vi "Lab14.vi"() -> ()   [LabVIEW 2022 SP3]
uses:
  <vilib>/DAQmx/create/channels.llb/DAQmx Create Channel (CO-Pulse Generation-Frequency).vi
  <vilib>/DAQmx/configure/timing.llb/DAQmx Timing (Implicit).vi
  <resource>/objmgr/daqmx.rc
panel:
  in  "Duty Cycle":dbl(slide)=0.01 min=0.01 max=0.99 step=0.01 scale=0.0..1.0
  out "Iteration Number":i32
  in  "CO.Pulse.Term":tag="/Dev1/PFI1"
  in  "stop":bool
  in  "Counter":tag="Dev1/ctr0"
  in  "Frequency":dbl(slide)=5000.0 min=1.0 max=25000000.0 step=1.0 scale=1.0..25000000.0 scale format="%#_6p"
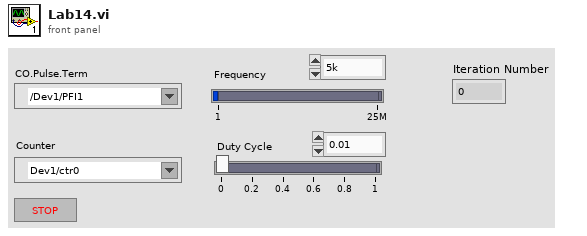
[diagram p1: front panel]
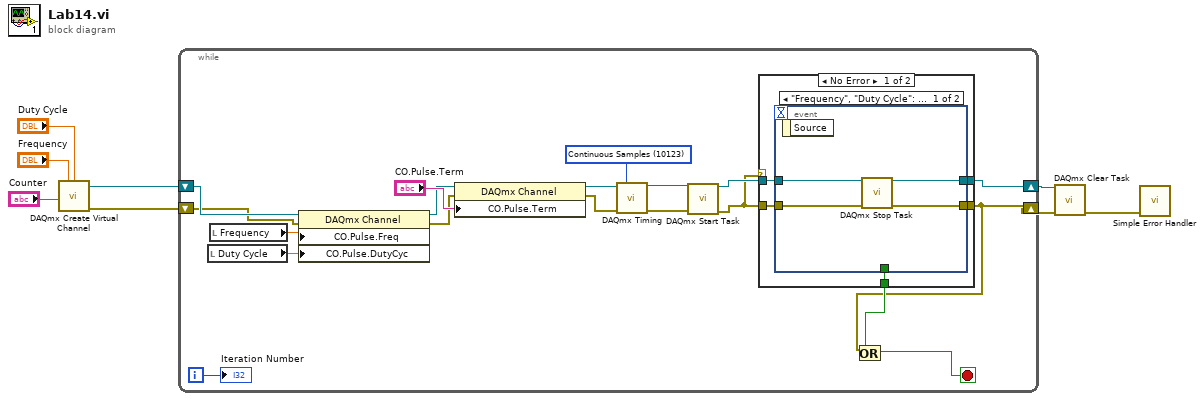
[diagram p0: block diagram]
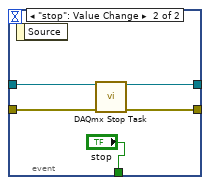
[diagram p2: hidden frame]
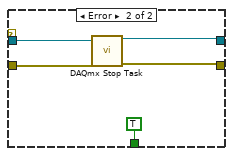
[diagram p3: hidden frame]
diagram:
  n1 = call-poly <vilib>:"DAQmx Create Virtual Channel.vi"("frequency"="Frequency", "duty cycle"="Duty Cycle", "counter"="Counter") -> ("task out"=w5:refnum<k21>, "error out"=w4:errorcluster)  [unwired: 11 in]
  n2 = while {
    shift-right: [w9] -> w2
    shift-left: w4 -> [w17]
    shift-right: [w20] -> w3
    shift-left: w5 -> [w18]
    i -> [w14]
    stop <- w11 stop-if-true
    w21 = 10123 items=["Finite Samples"=10178, "Continuous Samples"=10123, "Hardware Timed Single Point"=12522] ("sample mode")
    n3 = local read "Duty Cycle"() -> (w13:dbl)
    n4 = local read "Frequency"() -> (w19:dbl)
    n5 = property class="DAQmx Channel"(reference=w18, error in=w17, "CO.Pulse.Freq"=w19, "CO.Pulse.DutyCyc"=w13) -> (reference out=w16:refnum<k21>, error out=w15:errorcluster)
    n6 = property class="DAQmx Channel"(reference=w16, error in=w15, "CO.Pulse.Term"="CO.Pulse.Term") -> (reference out=w25:refnum<k21>, error out=w24:errorcluster)
    n7 = call-poly <vilib>:"DAQmx Timing.vi"("task/channels in"=w25, "sample mode"=w21, "error in"=w24) -> ("task out"=w23:refnum<k21>, "error out"=w22:errorcluster)  [unwired: 11 in]
    n8 = call <vilib>:"DAQmx Start Task.vi"("task/channels in"=w23, "error in"=w22) -> ("task out"=w27:refnum<k21>, "error out"=w10:errorcluster)  [unwired: 12 in]
    n9 = case shown="No Error" w10 {
      tunnel: w27 -> [w32 w46]
      tunnel: w10 -> [w31 w44]
      tunnel: [w30 w45] -> w20
      tunnel: [w29 w43] -> w9
      tunnel: [w28 TRUE ("stop")] -> w12
      frame No Error {
        n10 = event shown="[0] \"Frequency\", \"Duty Cycle\": Value Change" {
          selector: _ -> [_ _]
          dyn-events: _ -> [_ _]
          timeout: _ -> [_ _]
          tunnel: w32 -> [w36 w41]
          tunnel: w31 -> [w35 w40]
          tunnel: [w34 w38] -> w30
          tunnel: [w33 w39] -> w29
          tunnel: [_ "stop"] -> w28
          event "Frequency", "Duty Cycle": Value Change {
            n11 = event-data() -> ()  [unwired: 1 in, 1 out]
            n12 = call <vilib>:"DAQmx Stop Task.vi"("task/channels in"=w36, "error in"=w35) -> ("task out"=w34:refnum<k21>, "error out"=w33:errorcluster)  [unwired: 12 in]
          }
          event "stop": Value Change {
            n13 = event-data() -> ()  [unwired: 1 in, 1 out]
            n14 = call <vilib>:"DAQmx Stop Task.vi"("task/channels in"=w41, "error in"=w40) -> ("task out"=w38:refnum<k21>, "error out"=w39:errorcluster)  [unwired: 12 in]
          }
        }
      }
      frame Error {
        n15 = call <vilib>:"DAQmx Stop Task.vi"("task/channels in"=w46, "error in"=w44) -> ("task out"=w45:refnum<k21>, "error out"=w43:errorcluster)  [unwired: 12 in]
      }
    }
    n16 = Or(x=w9, y=w12) -> (x .or. y?=w11:bool)
    "Iteration Number" <- w14
  }
  n17 = call <vilib>:"DAQmx Clear Task.vi"("task in"=w3, "error in"=w2) -> ("error out"=w8:errorcluster)  [unwired: 13 in]
  n18 = call <vilib>:"Simple Error Handler.vi"("error in (no error)"=w8) -> ()  [unwired: 4 in, 5 out]
